vi "HTML-Generator-main.vi"(7 "tasks":T1[](array[typedef])=[{"State machine"=enum."add-red-box-header", "HTML before"="", "HTML after"=""}, {"State machine"=enum."Add VI description", "HTML before"="<h1>My Main Tool description</h1>\n<h2>Where it all began</h2> \n<br>", "HTML after"=""}, {"State machine"=enum."Add front panel", "HTML before"="<h1>Front Panel visible view</h1>\njust some text about the VI <br>", "HTML after"="<br>Picture text if one desires"}, {"State machine"=enum."Add Block Diagram", "HTML before"="<h1> Code</h1>\n<br>", "HTML after"=""}, {"State machine"=enum."Add VI hiearchy", "HTML before"="<h1>VI hiearchy</h1>\n<br>", "HTML after"=""}], 8 "error in":errorcluster, 9 "report file destination":path=path "/Macintosh HD/Users/oddoa/Work/LabVIEW/Vi-Documentation/generated", 11 "VI path":path=path "/Macintosh HD/Users/oddoa/Work/LabVIEW/Vi-Documentation/TestViProject/My Main VI.vi") -> (0 "error out":errorcluster)   [LabVIEW 2014]
uses:
  controls/state program.ctl
  controls/state-machine.ctl
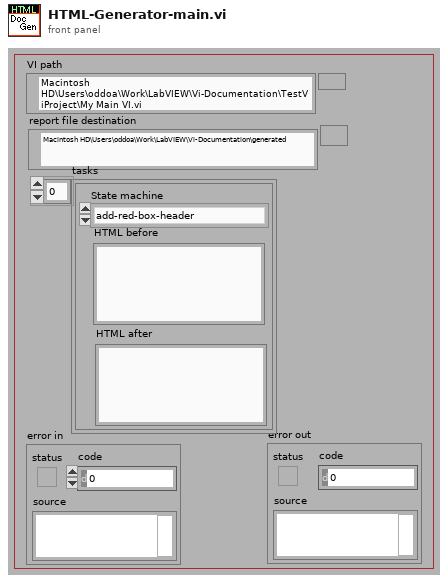
[diagram p1: front panel]
types:
  T1 = typedef "state program.ctl" = cluster{"State machine":T2, "HTML before":string, "HTML after":string}
  T2 = typedef "state-machine.ctl" = enum16{"add carridge return", "init", "Read-inputs", "edit generated file", "end", "Add front panel", "Add Block Diagram", "Add VI icon", "Add VI description", "Add VI hiearchy", "Add list of sub vis", "add custom html", "open report in browser", "Save report to file", "dispose report", "Add header text", "Create style .css", "add-red-box-header", "Delete Temp Files", "Remove-path-element", "add-revision-history", "add-icon-image-only"}
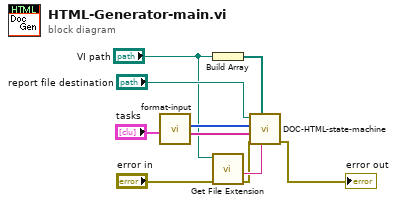
[diagram p0: block diagram]
diagram:
  n1 = call "format-input.vi"("tasks"="tasks") -> ("HTML"=w8:string[], "states"=w9:T2[])  [unwired: 9 out]
  n2 = Build Array("VI path") -> (w1:path[])
  n3 = call <vilib>:"Get File Extension.vi"("error in (no error)"="error in", "file"="VI path") -> ("error out"=w2:errorcluster, "filename without extension"=w3:string)  [unwired: 8 out]
  n4 = call "DOC-HTML-state-machine.vi"("header"=w3, "VI paths"=w1, "error in"=w2, "HTML"=w8, "states"=w9, "report file destination"="report file destination") -> ("error out"=→"error out":errorcluster)  [unwired: 3 in, 2 out]
